vi "GFITS_ImageFinished.vi"(0 "file reference":u64, 1 "multimple extensions":bool, 2 "_before_ expID":string, 3 "num of extensions":u16=16, 5 "nodeID":string, 6 "logfile":path, 7 "filemsg":string, 9 "image name":string, 10 "number of keywords":i32[](array[numeric]), 11 "error in (no error)":errorcluster, 12 "Database RefNum in":T1, 13 "headers":bool=TRUE, 14 "progress":i16) -> (4 "file reference out":u64, 8 "expID":string, 15 "error out":errorcluster)   [LabVIEW 2016]
uses:
  DBSHAND/private/vis/DatabaseHand_RefNum.ctl
  Common/public/vis/CMN_FVAR_action.ctl
  DBSHAND/private/vis/DatabaseHand_Element_Get(string).vi
panel:
  in  "Log":bool=TRUE
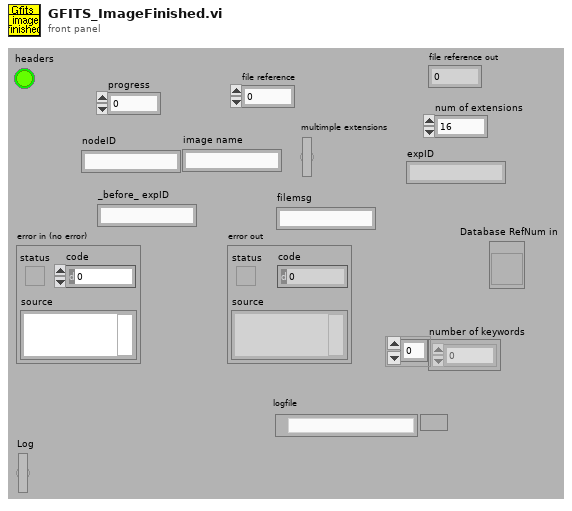
[diagram p1: front panel]
types:
  T1 = typedef "DatabaseHand_RefNum.ctl" = refnum<vi>
  T2 = typedef "CMN_FVAR_action.ctl" = enum16{"read", "write"}
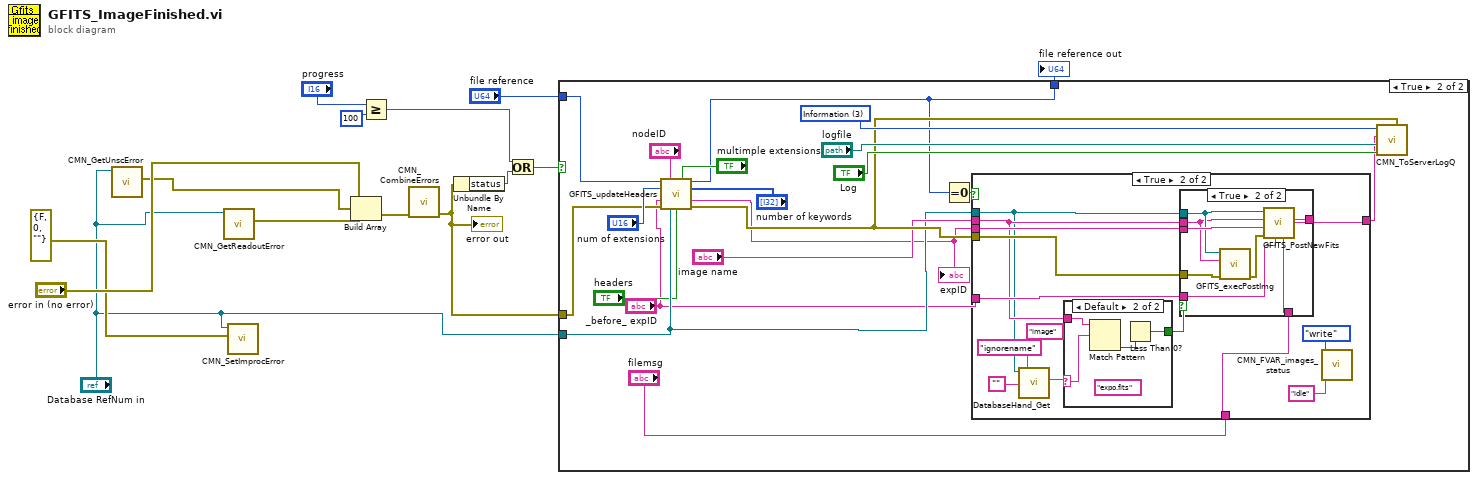
[diagram p0: block diagram]
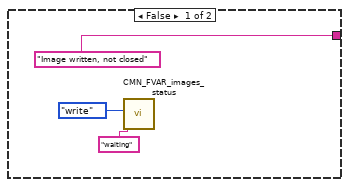
[diagram p3: hidden frame]
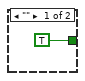
[diagram p4: hidden frame]
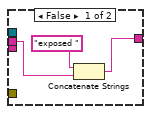
[diagram p5: hidden frame]
diagram:
  n1 = call "CMN_GetUnscError.vi"("Database RefNum in"="Database RefNum in") -> ("unsc_error"=w1:errorcluster)  [unwired: 1 in, 9 out]
  n2 = call "CMN_GetReadoutError.vi"("Database RefNum in"="Database RefNum in") -> ("readout_error"=w4:errorcluster)  [unwired: 1 in, 9 out]
  n3 = call "CMN_SetImprocError.vi"("improc error"=errorcluster {"status"=FALSE, "code"=0, "source"=""} ("error in (no error)"), "Database RefNum in"="Database RefNum in") -> ()  [unwired: 1 in, 9 out]
  n4 = Build Array("error in (no error)", w1, w4) -> (w12:errorcluster[])
  n5 = Greater Or Equal?(x="progress", y=u16 100) -> (x >= y?=w10:bool)
  n6 = call "CMN_CombineErrors.vi"("Errors"=w12) -> ("error out"=w8:errorcluster)  [unwired: 10 out]
  "error out" <- w8
  n7 = Unbundle By Name(w8) -> ("status"=w11:bool)
  n8 = Or(x=w10, y=w11) -> (x .or. y?=w9:bool)
  n9 = case shown="True" w9 {
    tunnel: w8 -> [_ w31]
    tunnel: "file reference" -> [w15 w30]
    tunnel: [w15 w17] -> w6
    tunnel: "Database RefNum in" -> [_ w23]
    frame False {
    }
    frame True {
      w29 = u16 3 items=["command", "imediateReply", "Callback Reply", "Information"] ("type")
      n10 = call "GFITS_updateHeaders.vi"("fref"=w30, "nodeID"="nodeID", "Multiple extensions?"="multimple extensions", "num of extensions"="num of extensions", "number of keywords"="number of keywords", "expID in"="_before_ expID", "error in (no error)"=w31, "Database RefNum in"=w23, "headers"="headers") -> ("ref out"=w17:u64, "expID"=w22:string, "error out"=w26:errorcluster)  [unwired: 4 out]
      "expID" <- w22
      n11 = Equal To 0?(x=w17) -> (x = 0?=w18:bool)
      n12 = case shown="True" w18 {
        tunnel: w26 -> [_ w46]
        tunnel: ["Image written, not closed" ("message") w50] -> w25
        tunnel: "image name" -> [_ w44]
        tunnel: w23 -> [_ w41]
        tunnel: w22 -> [_ w49]
        tunnel: "_before_ expID" -> [_ w45]
        tunnel: "filemsg" -> [_ w42]
        frame False {
          n13 = call "CMN_FVAR_images_status.vi"("value in"="waiting", "action"=CMN_FVAR_action."write") -> ()  [unwired: 9 out]
        }
        frame True {
          (unwired) "image" ("group")
          n14 = call-poly "DatabaseHand_Get.vi"("default value"="", "name"="ignorename", "Database RefNum in"=w41) -> ("value"=w38:string)  [unwired: 2 in, 6 out]
          n15 = case shown="Default" w38 {
            selector: w38 -> [_ w52]
            tunnel: w44 -> [_ w55]
            tunnel: [TRUE w53] -> w43
            frame "" {
            }
            frame Default {
              (unwired) "expo.fits" ("regular expression")
              n16 = Match Pattern(string=w55, regular expression=w52) -> (offset past match=w54:i32)  [unwired: 4 out]
              n17 = Less Than 0?(x=w54) -> (x < 0?=w53:bool)
            }
          }
          n18 = case shown="True" w43 {
            tunnel: [w56 w66] -> w50
            tunnel: w49 -> [_ w65]
            tunnel: w42 -> [_ w64]
            tunnel: w46 -> [_ w63]
            tunnel: w41 -> [_ w61]
            tunnel: w45 -> [_ w60]
            tunnel: w44 -> [w57 w59]
            frame False {
              n19 = Concatenate Strings("exposed " ("string"), w57) -> (w56:string)
            }
            frame True {
              n20 = call "GFITS_execPostImg.vi"("error in"=w63, "image name"=w59, "Database RefNum in"=w61) -> ("error out"=w62:errorcluster)  [unwired: 8 out]
              n21 = call "GFITS_PostNewFits.vi"("filemsg"=w64, "before_expID"=w60, "error in"=w62, "expID"=w65, "image name"=w59, "Database RefNum in"=w61) -> ("message"=w66:string)  [unwired: 5 out]
            }
          }
          n22 = call "CMN_FVAR_images_status.vi"("value in"="idle", "action"=CMN_FVAR_action."write") -> ()  [unwired: 9 out]
        }
      }
      n23 = call "CMN_ToServerLogQ.vi"("error in (no error)"=w26, "Log"="Log", "file"="logfile", "string"=w25, "type"=w29) -> ()  [unwired: 1 in, 5 out]
    }
  }
  "file reference out" <- w6
